vi "generate channels from UI.vi"(8 "error in":errorcluster, 11 "VI Refnum":refnum<vi>) -> (0 "error out":errorcluster, 3 "channels":refnum<class "TBM channel.lvclass">[](array[class]))   [LabVIEW 2013, in "UI Reference configuration.lvclass"]
uses:
  UI Reference configuration.lvclass
  <vilib>/NI/Tag Bus Module Framework/channel/TBM channel.lvclass
  <vilib>/NI/Tag Bus Module Framework/channel/channel classification.ctl
  <vilib>/NI/Tag Bus/tag/Data Type.ctl
  <vilib>/Utility/VariantDataType/VariantType.lvlib
  <vilib>/NI/Tag Bus/tag/tag descriptor.lvclass
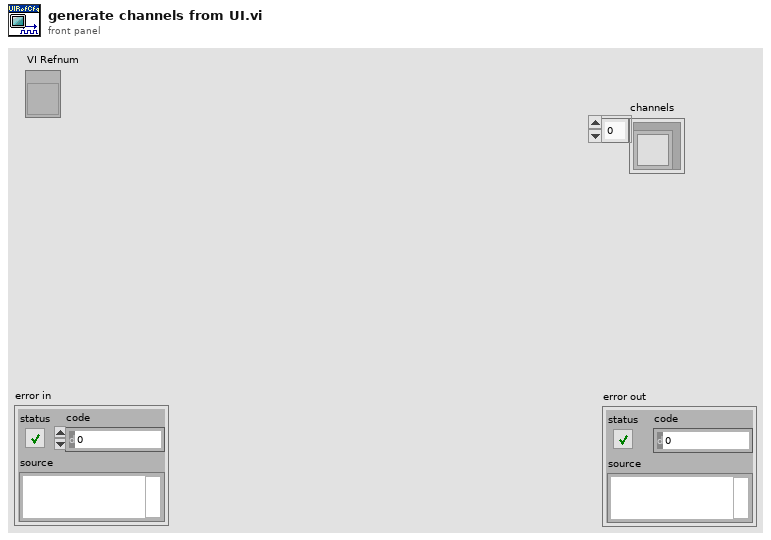
[diagram p1: front panel]
types:
  T1 = typedef "TBM channel.lvclass/channel classification.ctl" = enum16{"input data", "output data", "processing parameter", "processing result"}
  T2 = typedef "tag bus.lvlib/tag descriptor.lvclass/Data Type.ctl" = enum16{"Double", "Single", "I64", "I32", "I16", "I8", "U64", "U32", "U16", "U8", "Boolean", "String", "Array of Double", "Array of Single", "Array of I64", "Array of I32", "Array of I16", "Array of I8", "Array of U64", "Array of U32", "Array of U16", "Array of U8", "Array of Boolean", "Array of String"}
  T3 = typedef "VariantType.lvlib/Type.ctl" = enum8{"Invalid Type", "Void", "I8", "I16", "I32", "I64", "U8", "U16", "U32", "U64", "Single Float", "Double Float", "Extended Float", "Single Complex", "Double Complex", "Extended Complex", "Enum U8", "Enum U16", "Enum U32", "Enum U64", "Single Float With Unit", "Double Float With Unit", "Extended Float With Unit", "Single Complex with Unit", "Double Complex with Unit", "Extended Complex with Unit", "Boolean", "String", "Path", "Picture", "Tag", "Array", "Cluster", "Variant", "LV Variant", "Waveform", "Timestamp", "Digital Waveform", "Digital Data", "ExpressData", "Refnum", "External Data", "VI", "Poly VI", "LabVIEW Class Instance", "Fixed Point"}
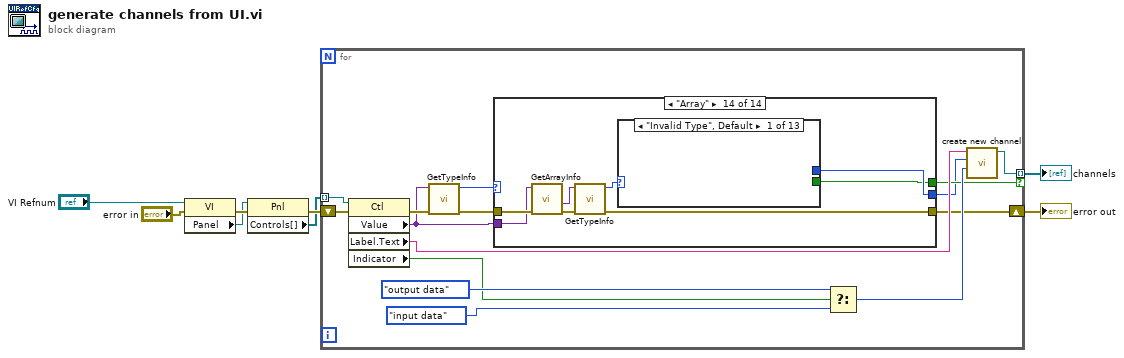
[diagram p0: block diagram]
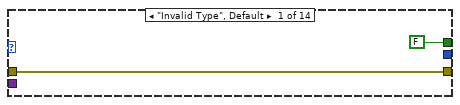
[diagram p2: hidden frame]
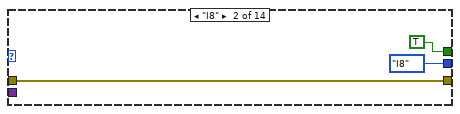
[diagram p3: hidden frame]
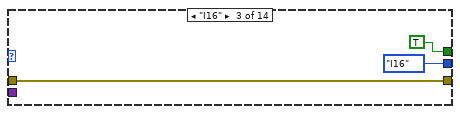
[diagram p4: hidden frame]
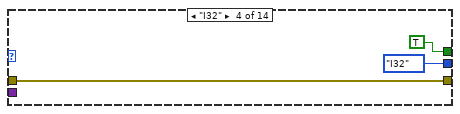
[diagram p5: hidden frame]
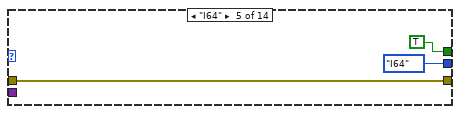
[diagram p6: hidden frame]
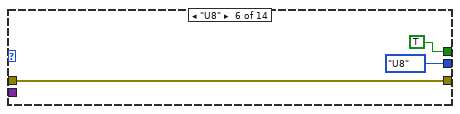
[diagram p7: hidden frame]
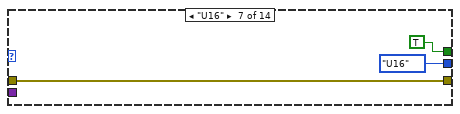
[diagram p8: hidden frame]
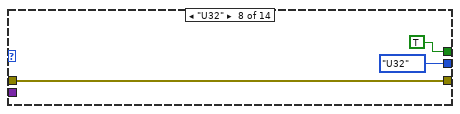
[diagram p9: hidden frame]
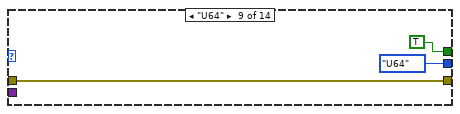
[diagram p10: hidden frame]
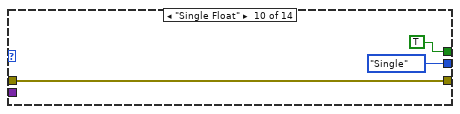
[diagram p11: hidden frame]
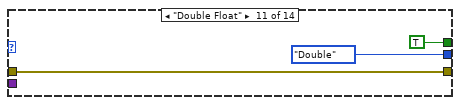
[diagram p12: hidden frame]
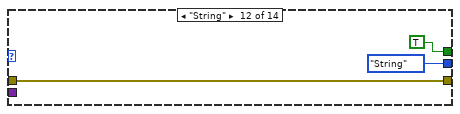
[diagram p13: hidden frame]
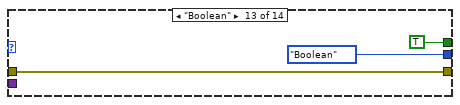
[diagram p14: hidden frame]
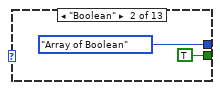
[diagram p15: hidden frame]
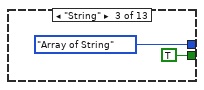
[diagram p16: hidden frame]
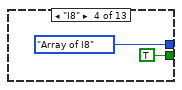
[diagram p17: hidden frame]
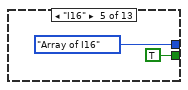
[diagram p18: hidden frame]
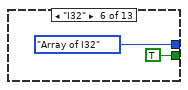
[diagram p19: hidden frame]
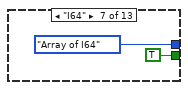
[diagram p20: hidden frame]
diagram:
  n1 = property class="VI"(reference="VI Refnum", error in="error in") -> (error out=w8:errorcluster, "Panel"=w7:refnum<vi>)  [unwired: 1 out]
  n2 = property class="Pnl"(reference=w7, error in=w8) -> (error out=w6:errorcluster, "Controls[]"=w5:refnum<vi>[])  [unwired: 1 out]
  n3 = for {
    shift-right: [w9] -> w2
    shift-left: w6 -> [w22]
    tunnel: w5 -> [w23] mode=indexing
    tunnel: [w21] -> w1 mode=indexing if=w11
    n4 = property class="Ctl"(reference=w23, error in=w22) -> (error out=w15:errorcluster, "Value"=w12:variant, "Label.Text"=w20:string, "Indicator"=w17:bool)  [unwired: 1 out]
    n5 = call <vilib>:"GetTypeInfo.vi"("error in (no error)"=w15, "Variant"=w12) -> ("error out"=w13:errorcluster, "Type Enum"=w14:T3)  [unwired: 5 in, 3 out]
    n6 = case shown="\"Array\"" w14 {
      tunnel: w13 -> [w24 w26 w29 w32 w35 w38 w41 w44 w47 w50 w53 w56 w59 w69]
      tunnel: w12 -> [_ _ _ _ _ _ _ _ _ _ _ _ _ w68]
      tunnel: [FALSE TRUE TRUE TRUE TRUE TRUE TRUE TRUE TRUE TRUE TRUE TRUE TRUE w62] -> w11
      tunnel: [_ Data_Type."I8" ("data type") Data_Type."I16" ("data type") Data_Type."I32" ("data type") Data_Type."I64" ("data type") Data_Type."U8" ("data type") Data_Type."U16" ("data type") Data_Type."U32" ("data type") Data_Type."U64" ("data type") Data_Type."Single" ("data type") Data_Type."Double" ("data type") Data_Type."String" ("data type") Data_Type."Boolean" ("data type") w63] -> w10
      tunnel: [w24 w26 w29 w32 w35 w38 w41 w44 w47 w50 w53 w56 w59 w65] -> w9
      frame "Invalid Type", Default {
      }
      frame "I8" {
      }
      frame "I16" {
      }
      frame "I32" {
      }
      frame "I64" {
      }
      frame "U8" {
      }
      frame "U16" {
      }
      frame "U32" {
      }
      frame "U64" {
      }
      frame "Single Float" {
      }
      frame "Double Float" {
      }
      frame "String" {
      }
      frame "Boolean" {
      }
      frame "Array" {
        n7 = call <vilib>:"GetArrayInfo.vi"("error in (no error)"=w69, "Variant"=w68) -> ("error out"=w67:errorcluster, "ArrayElement"=w66:variant)  [unwired: 6 in, 2 out]
        n8 = call <vilib>:"GetTypeInfo.vi"("error in (no error)"=w67, "Variant"=w66) -> ("error out"=w65:errorcluster, "Type Enum"=w64:T3)  [unwired: 5 in, 3 out]
        n9 = case shown="\"Invalid Type\", Default" w64 {
          tunnel: [_ Data_Type."Array of Boolean" ("data type") Data_Type."Array of String" ("data type") Data_Type."Array of I8" ("data type") Data_Type."Array of I16" ("data type") Data_Type."Array of I32" ("data type") Data_Type."Array of I64" ("data type") Data_Type."Array of U8" ("data type") Data_Type."Array of U16" ("data type") Data_Type."Array of U32" ("data type") Data_Type."Array of U64" ("data type") Data_Type."Array of Single" ("data type") Data_Type."Array of Double" ("data type")] -> w63
          tunnel: [_ TRUE TRUE TRUE TRUE TRUE TRUE TRUE TRUE TRUE TRUE TRUE TRUE] -> w62
          frame "Invalid Type", Default {
          }
          frame "Boolean" {
          }
          frame "String" {
          }
          frame "I8" {
          }
          frame "I16" {
          }
          frame "I32" {
          }
          frame "I64" {
          }
          frame "U8" {
          }
          frame "U16" {
          }
          frame "U32" {
          }
          frame "U64" {
          }
          frame "Single Float" {
          }
          frame "Double Float" {
          }
        }
      }
    }
    n10 = Select(t=channel_classification."output data" ("channel classification"), s=w17, f=channel_classification."input data" ("channel classification")) -> (s? t:f=w16:T1)
    n11 = call <vilib>:"create new channel.vi"("channel classification"=w16, "data type"=w10, "channel name"=w20) -> ("channel"=w21:refnum<class "TBM channel.lvclass">)  [unwired: 8 in]
  }
  "error out" <- w2
  "channels" <- w1
